vi "read_occupancy.vi"() -> ()   [LabVIEW 2011]
uses:
  Dependencies/global.vi
panel:
  out "Events":u32[][](array[numeric])
  out "Reset":bool=TRUE
  in  "Reset to Number:":dbl
  in  "Reset Counter":bool
  in  "Reset at:":string="00:00:00"
  out "Current Time":string
  out "Occupancy":dbl(graph)
  out "element":string
  out "Deque error":errorcluster
  out "DataSocket error":errorcluster
  out "# Sent Data":u64
  out "The number of people inside A:225:":dbl
  in  "Initial number of people inside A:225:":dbl
  out "Estimated events":dbl[](array[numeric])
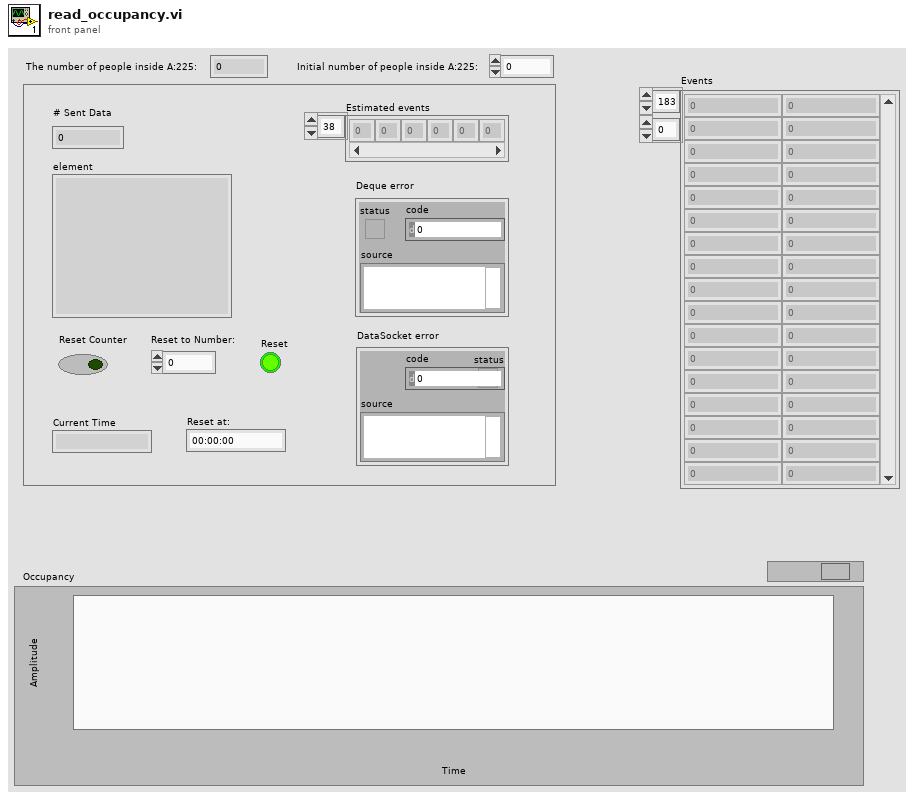
[diagram p1: front panel]
types:
  T1 = enum16{"Read", "Write", "ReadWrite", "BufferedRead", "BufferedReadWrite"}
  T2 = typedef "imagedata.ctl" = cluster{"image type":i32, "image depth":i32, "image":u8[], "mask":u8[], "colors":u32[], "Rectangle":cluster{"left":i16, "top":i16, "right":i16, "bottom":i16}}
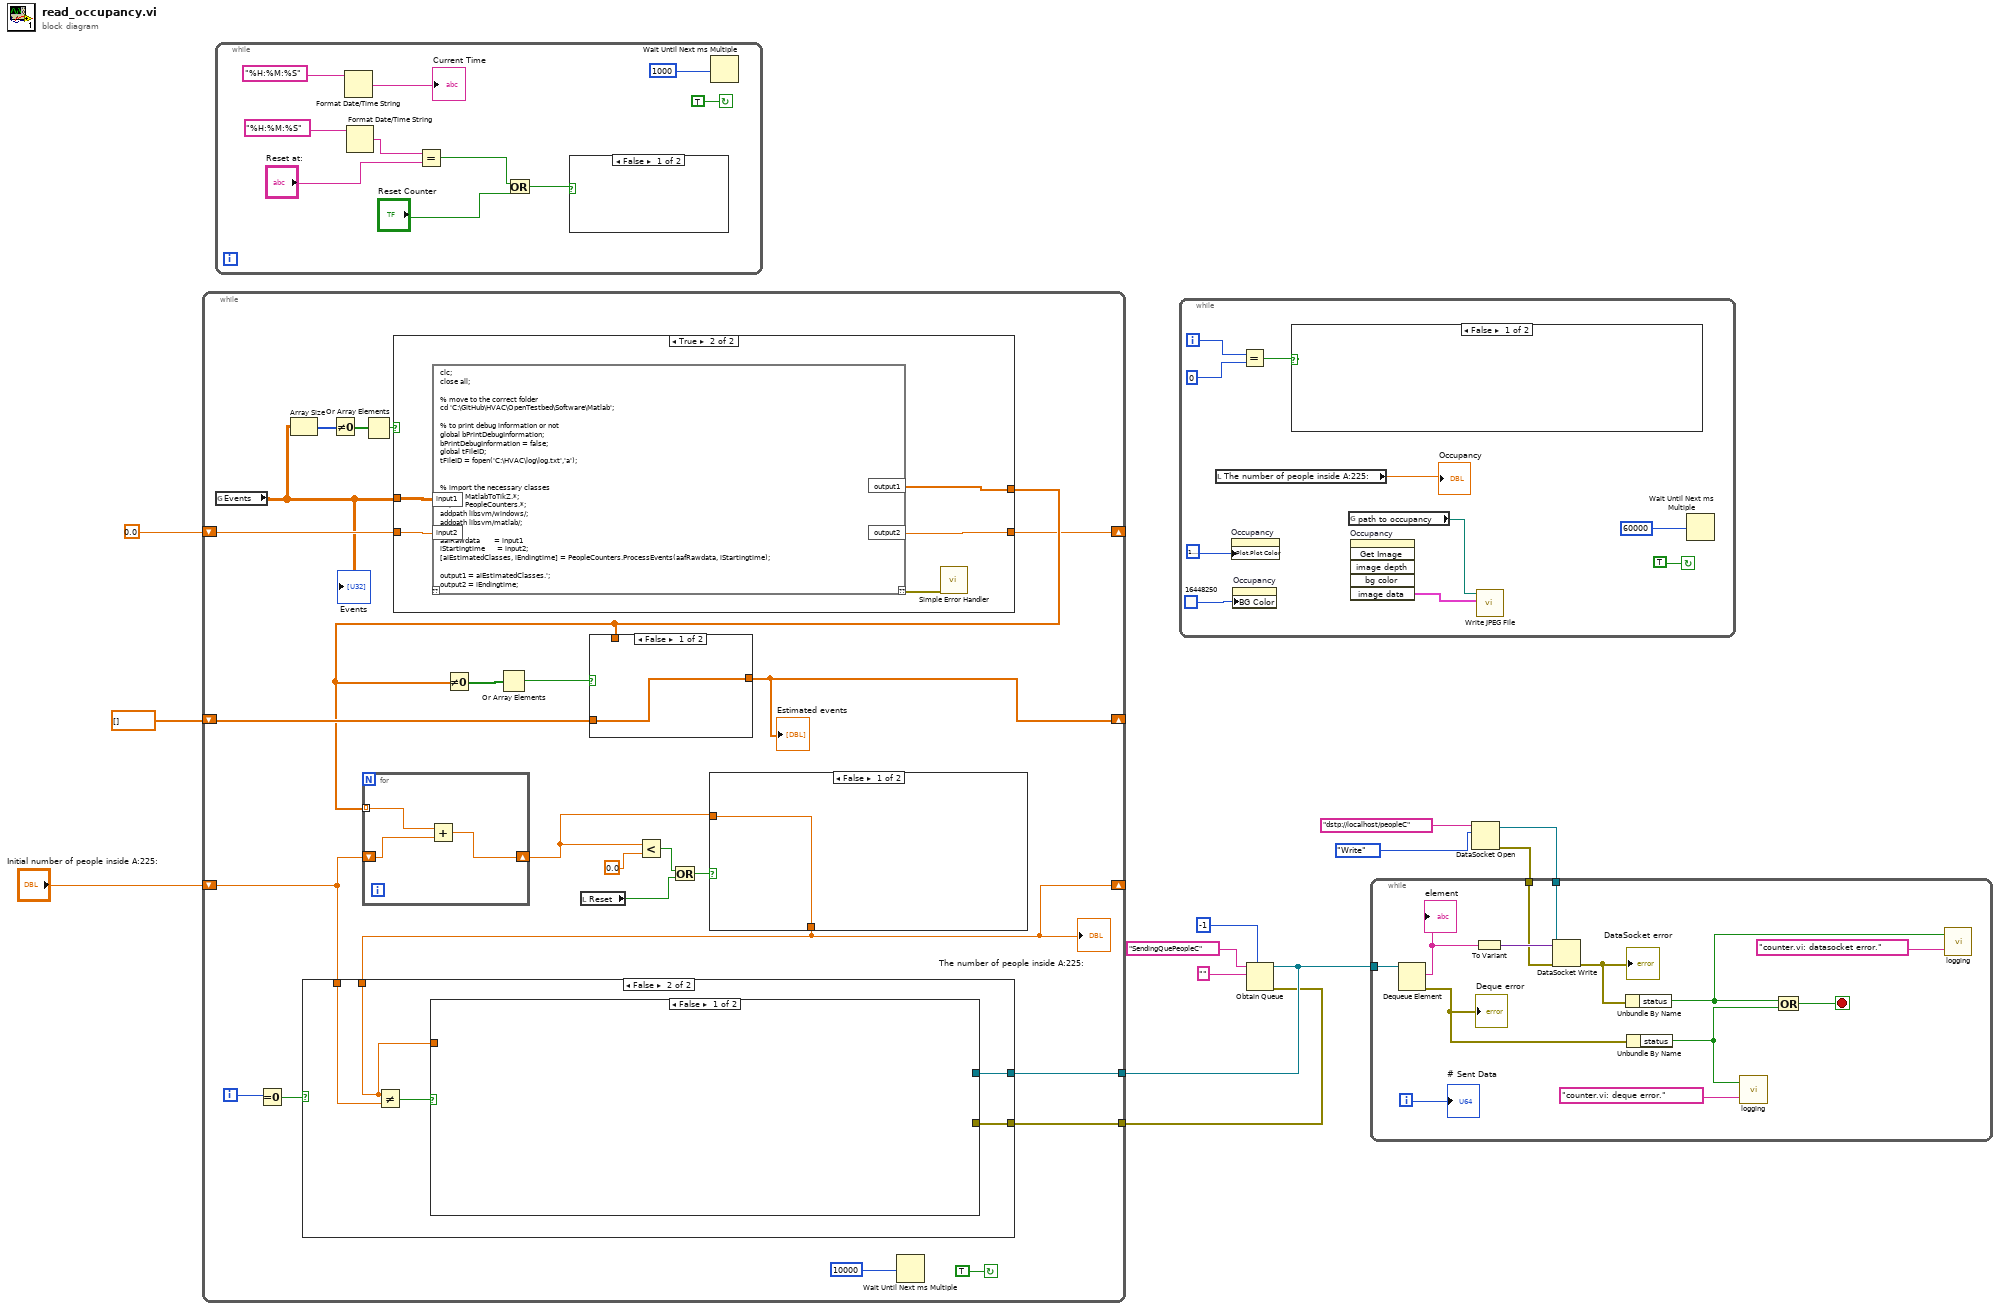
[diagram p0: block diagram]
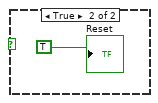
[diagram p2: hidden frame]
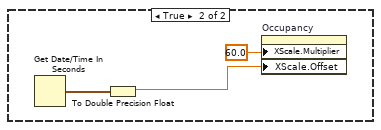
[diagram p3: hidden frame]
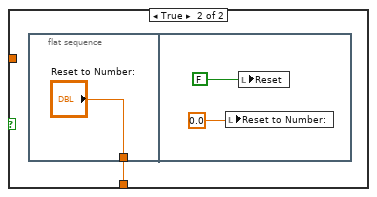
[diagram p4: hidden frame]
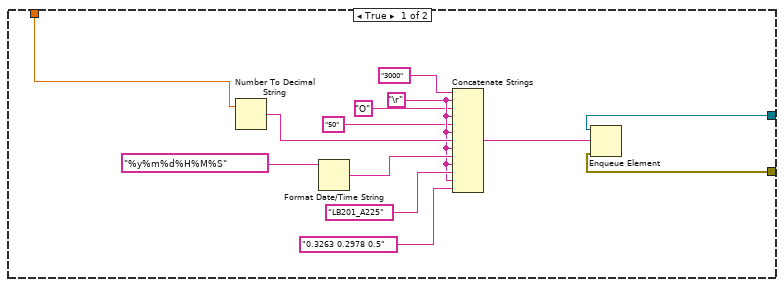
[diagram p5: hidden frame]
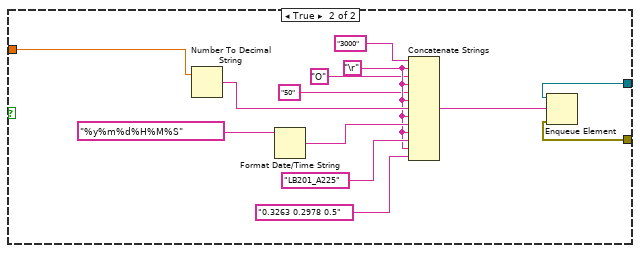
[diagram p6: hidden frame]
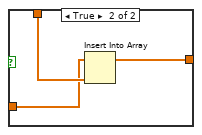
[diagram p7: hidden frame]
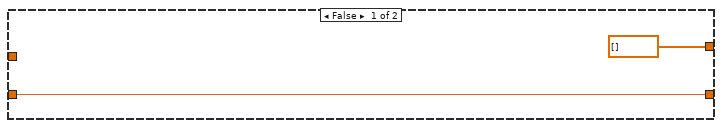
[diagram p8: hidden frame]
diagram:
  n1 = while {
    stop <- TRUE continue-if-true
    n2 = Format Date/Time String(time format string (%c)="%H:%M:%S") -> (date/time string=→"Current Time":string)  [unwired: 2 in]
    n3 = Format Date/Time String(time format string (%c)="%H:%M:%S") -> (date/time string=w19:string)  [unwired: 2 in]
    n4 = Equal?(x=w19, y="Reset at:") -> (x = y?=w15:bool)
    n5 = Or(x=w15, y="Reset Counter") -> (x .or. y?=w14:bool)
    n6 = case shown="False" w14 {
      frame False {
      }
      frame True {
        "Reset" <- TRUE ("Reset Counter")
      }
    }
    n7 = Wait Until Next ms Multiple(millisecond multiple=u32 1000 ("milliseconds to wait")) -> ()  [unwired: 1 out]
  }
  n8 = while {
    i -> [w30]
    stop <- TRUE continue-if-true
    n9 = local read "The number of people inside A:225:"() -> (→"Occupancy":dbl)
    n10 = property on="Occupancy" class="WFChart (strict)"("Plot.Plot Color"=u32 16777222) -> ()  [unwired: 2 in, 2 out]
    n11 = property on="Occupancy" class="WFChart (strict)"("BG Color"=u32 16448250) -> ()  [unwired: 2 in, 2 out]
    n12 = Equal?(x=w30, y=i16 0) -> (x = y?=w32:bool)
    n13 = case shown="False" w32 {
      frame False {
      }
      frame True {
        n14 = Get Date/Time In Seconds() -> (seconds since 1Jan1904=w36:timestamp)
        n15 = To Double Precision Float(number=w36) -> (double precision float=w35:dbl)
        n16 = property on="Occupancy" class="WFChart (strict)"("XScale.Multiplier"=60.0 ("X Scale.Offset and Multiplier:Multiplier"), "XScale.Offset"=w35) -> ()  [unwired: 2 in, 2 out]
      }
    }
    n17 = global read "global.vi" "path to occupancy"() -> (w26:path)
    n18 = invoke on="Occupancy" class="WFChart (strict)" method="Get Image"() -> ("image data"=w27:T2)  [unwired: 6 in, 5 out]
    n19 = call <vilib>:"Write JPEG File.vi"("image data"=w27, "path to JPEG file"=w26) -> ()  [unwired: 8 in, 2 out]
    n20 = Wait Until Next ms Multiple(millisecond multiple=u32 60000 ("milliseconds to wait")) -> ()  [unwired: 1 out]
  }
  n21 = Obtain Queue(max queue size (-1, unlimited)=-1, name (unnamed)="SendingQuePeopleC", element data type="") -> (queue out=w5:refnum<queue>, error out=w4:errorcluster)  [unwired: 2 in, 1 out]
  n22 = while {
    shift-right: [w50] -> _
    shift-left: 0.0 ("Real Matrix Element") -> [w59]
    shift-right: [w51] -> _
    shift-left: dbl[] [] -> [w58]
    shift-right: [w37] -> _
    shift-left: "Initial number of people inside A:225:" -> [w48]
    tunnel: w5 -> [w47]
    tunnel: w4 -> [w46]
    i -> [w45]
    stop <- TRUE continue-if-true
    n23 = global read "global.vi" "Events"() -> (w43:dbl[][])
    "Events" <- w43
    n24 = Equal To 0?(x=w45) -> (x = 0?=w44:bool)
    n25 = Array Size(array=w43) -> (size(s)=w57:i32[])
    n26 = Not Equal To 0?(x=w57) -> (x != 0?=w56:bool[])
    n27 = Or Array Elements(Boolean array=w56) -> (logical OR=w55:bool)
    n28 = case shown="True" w55 {
      tunnel: w59 -> [w104 w110]
      tunnel: [w104 w109] -> w50
      tunnel: [dbl[] [] w108] -> w52
      tunnel: w43 -> [_ w107]
      frame False {
      }
      frame True {
        n29 = script code="clc;\nclose all;\n\n% move to the correct folder\ncd 'C:\\GitHub\\HVAC\\OpenTestbed\\Software\\Matlab';\n\n% to print debug information or not\nglobal bPrintDebugInformation;\nbPrintDebugInformation = false;\nglobal tFileID;\ntFileID = fopen('C:\\HVAC\\log\\log.txt','a');\n\n\n% import the necessary classes\nimport MatlabToTikZ.*;\nimport PeopleCounters.*;\naddpath libsvm/windows/;\naddpath libsvm/matlab/;\n\naafRawdata       = input1\niStartingtime      = input2;\n[aiEstimatedClasses, iEndingtime] = PeopleCounters.ProcessEvents(aafRawdata, iStartingtime);\n\noutput1 = aiEstimatedClasses.';\noutput2 = iEndingtime;"("input1"=w107, "input2"=w110) -> ("??"=w106:errorcluster, "output1"=w108:dbl[], "output2"=w109:dbl)  [unwired: 1 in]
        n30 = call <vilib>:"Simple Error Handler.vi"("error in (no error)"=w106) -> ()  [unwired: 4 in, 5 out]
      }
    }
    n31 = for {
      tunnel: w52 -> [w99] mode=indexing
      shift-right: [w97] -> w41
      shift-left: w48 -> [w98]
      n32 = Add(x=w99, y=w98) -> (x+y=w97:dbl)
    }
    n33 = Not Equal To 0?(x=w52) -> (x != 0?=w54:bool[])
    n34 = Or Array Elements(Boolean array=w54) -> (logical OR=w53:bool)
    n35 = local read "Reset"() -> (w38:bool)
    n36 = case shown="False" w53 {
      tunnel: w52 -> [_ w103]
      tunnel: w58 -> [w100 w102]
      tunnel: [w100 w101] -> w51
      frame False {
      }
      frame True {
        n37 = Insert Into Array(array=w102, new element=w103) -> (w101:dbl[])  [unwired: 1 in]
      }
    }
    "Estimated events" <- w51
    n38 = Less?(x=w41, y=0.0) -> (x < y?=w40:bool)
    n39 = Or(x=w40, y=w38) -> (x .or. y?=w39:bool)
    n40 = case shown="False" w39 {
      tunnel: w41 -> [w61 _]
      tunnel: [w61 w62] -> w37
      frame False {
      }
      frame True {
        n41 = flat-sequence {
          tunnel: ["Reset to Number:"] -> w62
          frame #0 {
          }
          frame #1 {
            n42 = local write "Reset to Number:"(0.0 ("Reset to Number:")) -> ()
            n43 = local write "Reset"(FALSE ("Reset")) -> ()
          }
        }
      }
    }
    "The number of people inside A:225:" <- w37
    n44 = case shown="False" w44 {
      tunnel: w37 -> [w66 w82]
      tunnel: w48 -> [_ w81]
      tunnel: w47 -> [w68 w80]
      tunnel: w46 -> [w67 w79]
      frame True {
        w73 = "\r"
        n45 = Number To Decimal String(number=w66) -> (decimal integer string=w77:string)  [unwired: 1 in]
        n46 = Format Date/Time String(time format string (%c)="%y%m%d%H%M%S") -> (date/time string=w75:string)  [unwired: 2 in]
        n47 = Concatenate Strings("3000" ("string"), w73, "O" ("string"), w73, "50" ("string"), w73, w77, w73, w75, w73, "LB201_A225", w73, "0.3263 0.2978 0.5" ("string")) -> (w69:string)
        n48 = Enqueue Element(queue=w68, element=w69, error in (no error)=w67) -> ()  [unwired: 1 in, 3 out]
      }
      frame False {
        n49 = Not Equal?(x=w82, y=w81) -> (x != y?=w83:bool)
        n50 = case shown="False" w83 {
          tunnel: w80 -> [_ w86]
          tunnel: w79 -> [_ w85]
          tunnel: w82 -> [_ w84]
          frame False {
          }
          frame True {
            w91 = "\r"
            n51 = Number To Decimal String(number=w84) -> (decimal integer string=w95:string)  [unwired: 1 in]
            n52 = Format Date/Time String(time format string (%c)="%y%m%d%H%M%S") -> (date/time string=w93:string)  [unwired: 2 in]
            n53 = Concatenate Strings("3000" ("string"), w91, "O" ("string"), w91, "50" ("string"), w91, w95, w91, w93, w91, "LB201_A225", w91, "0.3263 0.2978 0.5" ("string")) -> (w87:string)
            n54 = Enqueue Element(queue=w86, element=w87, error in (no error)=w85) -> ()  [unwired: 1 in, 3 out]
          }
        }
      }
    }
    n55 = Wait Until Next ms Multiple(millisecond multiple=u32 10000 ("milliseconds to wait")) -> ()  [unwired: 1 out]
  }
  n56 = DataSocket Open(10:T1."Write" ("mode"), 11:"dstp://localhost/peopleC" ("URL 3")) -> (0:w12:errorcluster, 3:w11:refnum<k13>)  [unwired: 2 in]
  n57 = while {
    tunnel: w5 -> [w123]
    tunnel: w11 -> [w122]
    tunnel: w12 -> [w118]
    i -> [w116]
    stop <- w117 stop-if-true
    n58 = Dequeue Element(queue=w123) -> (element=w111:string, error out=w120:errorcluster)  [unwired: 2 in, 2 out]
    "Deque error" <- w120
    "element" <- w111
    n59 = To Variant(anything=w111) -> (Variant=w121:variant)
    n60 = DataSocket Write(8:w118, 10:w121, 11:w122) -> (0:w119:errorcluster)  [unwired: 3 out]
    "DataSocket error" <- w119
    n61 = Unbundle By Name(w119) -> ("status"=w112:bool)
    n62 = Unbundle By Name(w120) -> ("status"=w114:bool)
    n63 = call "logging.vi"("data"="counter.vi: deque error.", "Boolean"=w114) -> ()  [unwired: 1 in]
    n64 = Compound Arithmetic op=OR(w112, w114) -> (w117:bool)
    n65 = call "logging.vi"("data"="counter.vi: datasocket error.", "Boolean"=w112) -> ()  [unwired: 1 in]
    "# Sent Data" <- w116
  }
